vi "[RT]NTC_Temp.vi"() -> (3 "Temp_NTC":dbl)   [LabVIEW 2018]
uses:
  <vilib>/myRIO/Common/Instrument Driver Framework/Utilities/typedefs/Analog Scaling Constants.ctl
  <vilib>/myRIO/Common/Instrument Driver Framework/Utilities/typedefs/Analog Scaling Constants List.ctl
  <vilib>/myRIO/Common/Instrument Driver Framework/myRIO v1.0/AI/typedefs/AI Channels Enum.ctl
  <vilib>/myRIO/Common/Instrument Driver Framework/myRIO v1.0/AI/typedefs/AI Channels List.ctl
  <vilib>/myRIO/Common/Instrument Driver Framework/Utilities/typedefs/Generic FPGA Reference.ctl
  <vilib>/myRIO/Common/Instrument Driver Framework/Utilities/typedefs/myRIO v1.0 Reference.ctl
  <vilib>/myRIO/Common/Instrument Driver Framework/Utilities/typedefs/Hardware Version Enum.ctl
  <vilib>/myRIO/Common/Instrument Driver Framework/Utilities/typedefs/myRIO Generic Hardware Reference.ctl
  <vilib>/myRIO/Instrument Drivers/Onboard IO/AI/typedefs/AI Reference.ctl
  <vilib>/myRIO/Instrument Drivers/Onboard IO/AI/AI.lvlib
  <vilib>/myRIO/Instrument Drivers/Onboard IO/AI/vis/myRIO AI Open.xnode
  <vilib>/myRIO/Common/Instrument Driver Framework/myRIO v1.0/AI/vis/myRIO v1.1 Open AI.vi
  <vilib>/userdefined/High Color/nirio_resource_hc.ctl
  [GlobVar]SensorState.vi
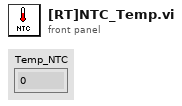
[diagram p1: front panel]
types:
  T1 = typedef "AI.lvlib/AI Reference.ctl" = cluster{"myRIO Reference":T2, "AI Channels List":T6, "AI Scaling Constants List":T8}
  T2 = typedef "myRIO Generic Hardware Reference.ctl" = cluster{"myRIO Model":T3, "myRIO Hardware Reference":T4}
  T3 = typedef "Hardware Version Enum.ctl" = enum16{"Unknown", "myRIO-1900", "myRIO-1950", "roboRIO", "NI ELVIS RIO CM", "ELVIS III"}
  T4 = typedef "myRIO v1.0 Reference.ctl" = cluster{"Generic FPGA Reference":T5, "Allow multiple opens":bool}
  T5 = typedef "Generic FPGA Reference.ctl" = refnum<k20>
  T6 = typedef "AI Channels List.ctl" = T7[]
  T7 = typedef "AI Channels Enum.ctl" = enum16{"Not Connected", "AudioIn/Left", "AudioIn/Right", "C/AI0", "C/AI1", "A/AI0", "A/AI1", "A/AI2", "A/AI3", "A/AI4", "A/AI5", "A/AI6", "A/AI7", "B/AI0", "B/AI1", "B/AI2", "B/AI3", "B/AI4", "B/AI5", "B/AI6", "B/AI7", "AI/AI0", "AI/AI1", "AI/AI2", "AI/AI3", "A/AI0 (DIFF)", "A/AI1 (DIFF)", "A/AI2 (DIFF)", "A/AI3 (DIFF)", "B/AI0 (DIFF)", "B/AI1 (DIFF)", "B/AI2 (DIFF)", "B/AI3 (DIFF)"}
  T8 = typedef "Analog Scaling Constants List.ctl" = T9[]
  T9 = typedef "Analog Scaling Constants.ctl" = cluster{"LSB Weight (Volts)":dbl, "Offset (Volts)":dbl, "Signed?":bool}
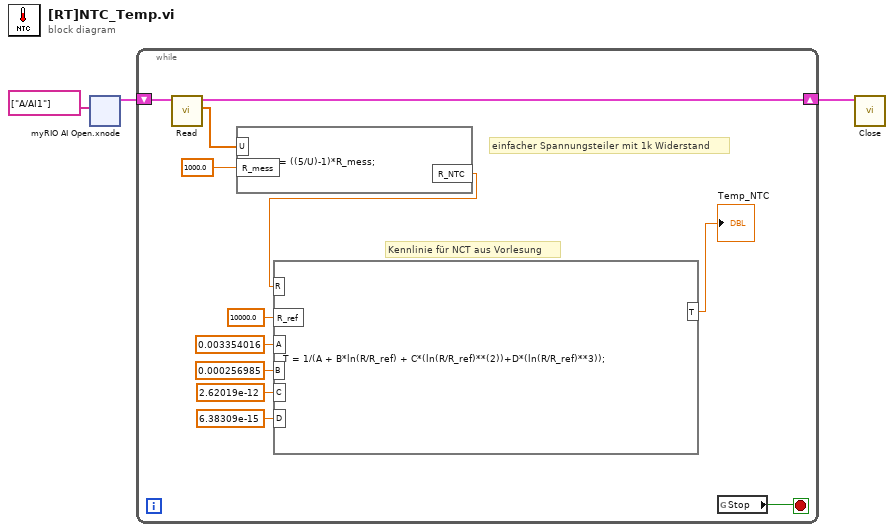
[diagram p0: block diagram]
diagram:
  n1 = xnode "myRIO AI Open.xnode"("Channel Names"=tag[] ["A/AI1"]) -> ("AI Ref Out"=w2:T1)  [unwired: 2 in, 1 out]
  n2 = while {
    shift-right: [w14] -> w1
    shift-left: w2 -> [w15]
    stop <- w4 stop-if-true
    # "einfacher Spannungsteiler mit 1k Widerstand"
    # "Kennlinie für NCT aus Vorlesung"
    n3 = call <vilib>:"Read.vi"("AI Ref In"=w15) -> ("Values"=w5:dbl[], "AI Ref Out"=w14:T1)  [unwired: 8 in, 1 out]
    n4 = formula code="R_NTC = ((5/U)-1)*R_mess;"("U"=w5, "R_mess"=1000.0 ("input variable")) -> ("R_NTC"=w12:dbl)
    n5 = formula code="T = 1/(A + B*ln(R/R_ref) + C*(ln(R/R_ref)**(2))+D*(ln(R/R_ref)**3));"("R_ref"=10000.0 ("input variable"), "R"=w12, "A"=0.003354016 ("input variable"), "B"=0.000256985 ("input variable"), "C"=2.62019e-12 ("input variable"), "D"=6.38309e-15 ("input variable")) -> ("T"=→"Temp_NTC":dbl)
    n6 = global read "[GlobVar]SensorState.vi" "Stop"() -> (w4:bool)
  }
  n7 = call <vilib>:"Close.vi"("AI Ref In"=w1) -> ()  [unwired: 10 in, 1 out]
